vi "Rozbijanie_NMEA_v1.1.vi"() -> ()   [LabVIEW 2014]
uses:
  <vilib>/Instr/_visa.llb/VISA Configure Serial Port (Instr).vi
  <vilib>/robotics/Protocols/NMEA/NMEA API.lvlib
panel:
  out "dane gpsa":T1 {"latitude" format="%#_10g"; "longitiude" format="%#_10g"}
  in  "stop udp":bool
  in  "udp 1":bool
  out "latitude (deg)":dbl format="%#_8g"
  out "longitude (deg)":dbl format="%#_8g"
  out "Cluster":T2 {"Latitude"."DD" format="%#_10g"; "Longitude"."DD" format="%#_10g"}
  out "GPS data":T3 {"oldest read timestamp" format="%^<%.3X\n%x>T"; "latitude (deg)" format="%#_10g"; "longitude (deg)" format="%#_10g"}
  out "f":string
  out "Sekundy 6":dbl
  out "Minuty 6":dbl
  out "Stopnie 6":ext
  out "Sekundy 5":dbl
  out "Minuty 5":dbl
  out "Stopnie 5":ext
  out "Sekundy 4":dbl
  out "Minuty 4":dbl
  out "Stopnie 4":ext
  out "Sekundy 3":dbl
  out "Minuty 3":dbl
  out "Stopnie 3":ext
  in  "stop":bool
  out "return count":u32
  in  "VISA resource name":refnum<visa-resource-name>="COM1"
  out "Sekundy 2":dbl
  out "Minuty 2":dbl
  out "Stopnie 2":ext
  out "Sekundy":dbl
  out "Minuty":dbl
  out "Stopnie":ext
  out "Array":string[](array[string])
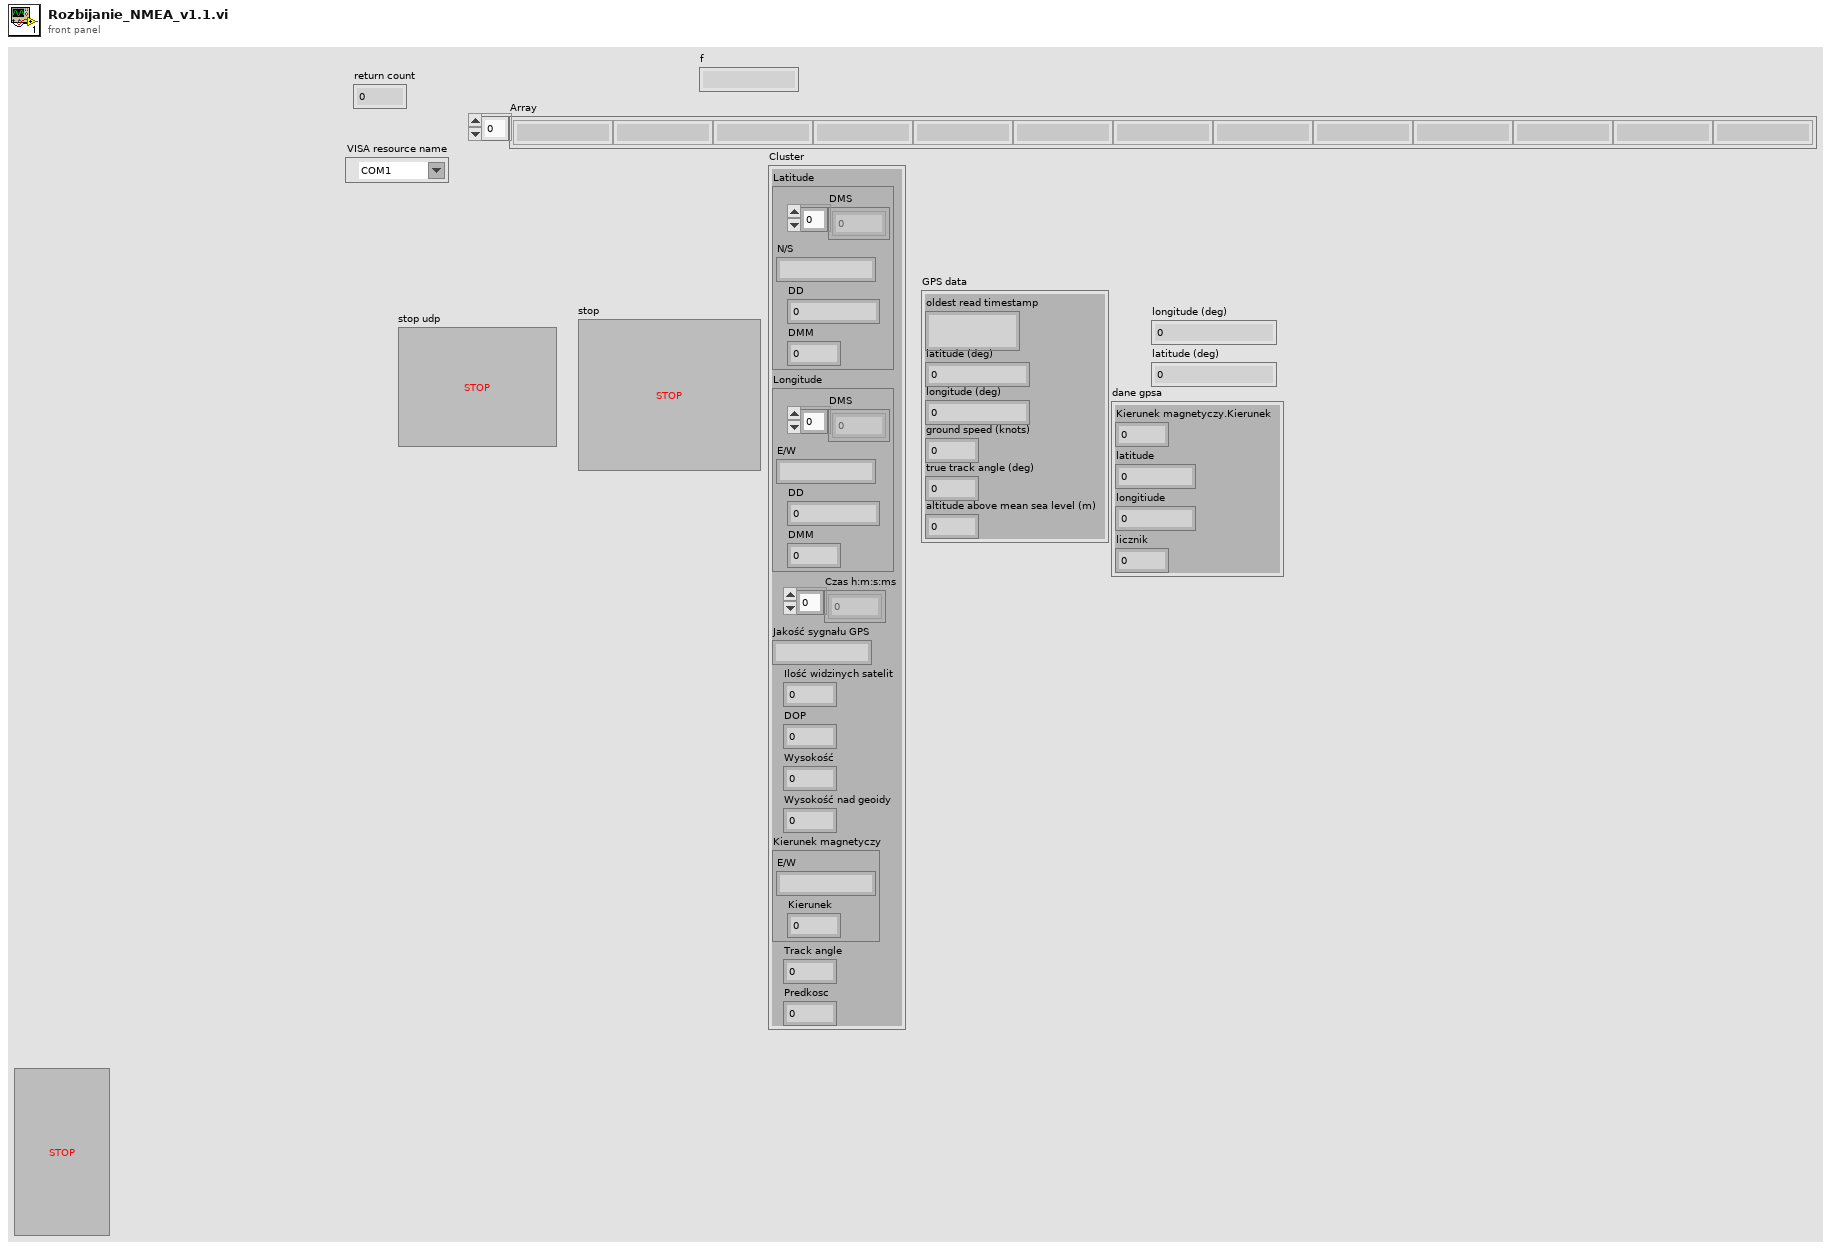
[diagram p1: front panel]
types:
  T1 = cluster{"Kierunek magnetyczy.Kierunek":dbl, "latitude":dbl, "longitiude":dbl, "licznik":dbl}
  T2 = cluster{"Latitude":cluster{"DMS":i32[], "N/S":string, "DD":dbl, "DMM":dbl}, "Longitude":cluster{"DMS":i32[], "E/W":string, "DD":dbl, "DMM":dbl}, "Czas h:m:s:ms":dbl[], "Jakość sygnału GPS":string, "Ilość widzinych satelit":i32, "DOP":dbl, "Wysokość":dbl, "Wysokość nad geoidy":dbl, "Kierunek magnetyczy":cluster{"E/W":string, "Kierunek":dbl}, "Track angle":dbl, "Predkosc":dbl}
  T3 = cluster{"oldest read timestamp":timestamp, "latitude (deg)":dbl, "longitude (deg)":dbl, "ground speed (knots)":dbl, "true track angle (deg)":dbl, "altitude above mean sea level (m)":dbl}
  T4 = cluster{"DMS":i32[], "E/W":string, "DD":dbl, "DMM":dbl}
  T5 = cluster{"DMS":i32[], "N/S":string, "DD":dbl, "DMM":dbl}
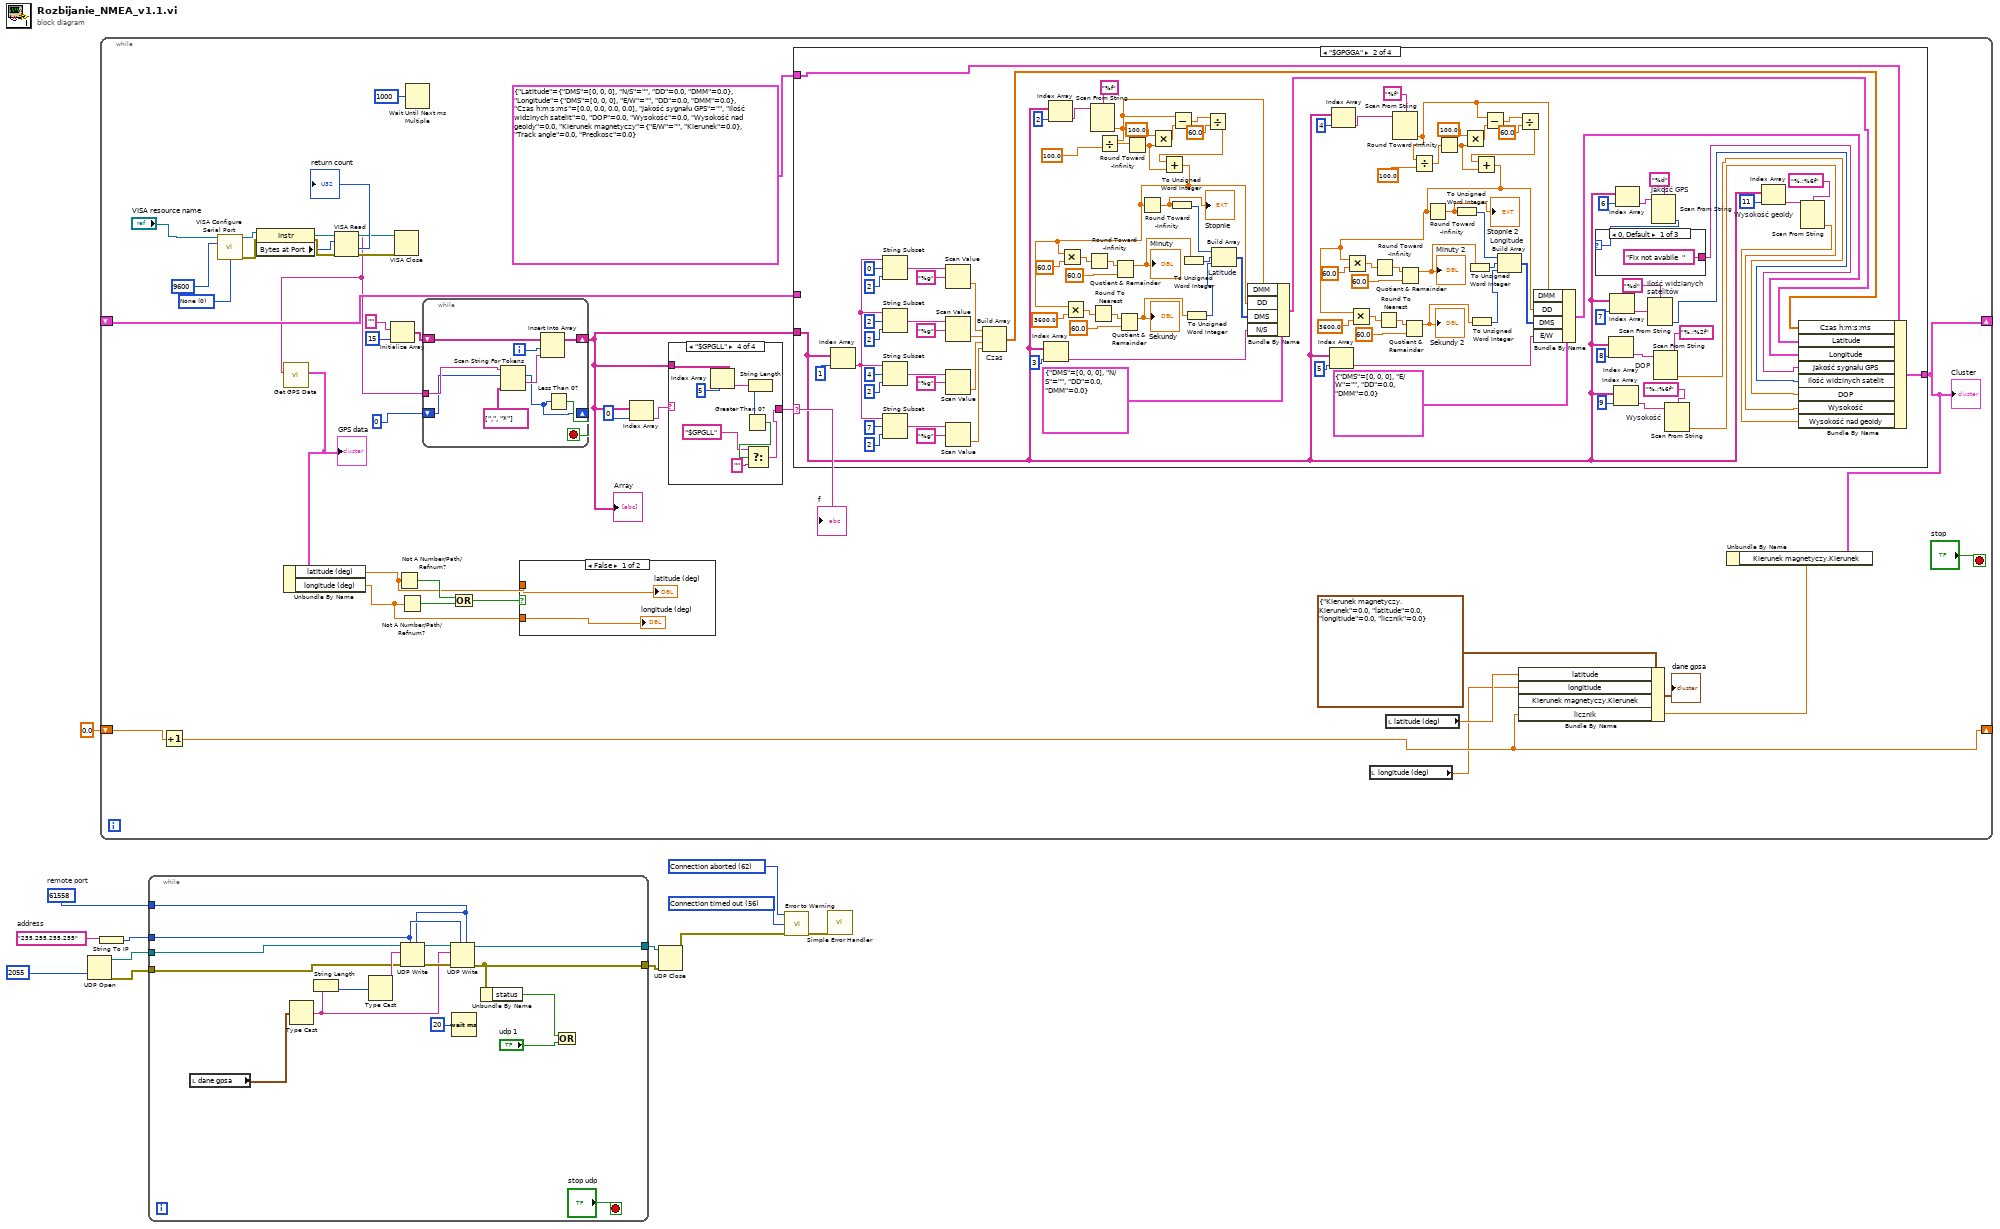
[diagram p0: block diagram]
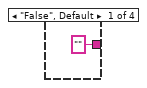
[diagram p3: hidden frame]
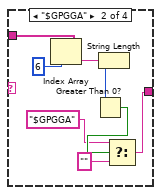
[diagram p4: hidden frame]
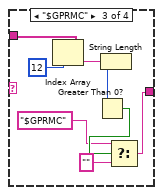
[diagram p5: hidden frame]
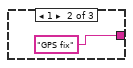
[diagram p7: hidden frame]
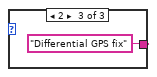
[diagram p8: hidden frame]
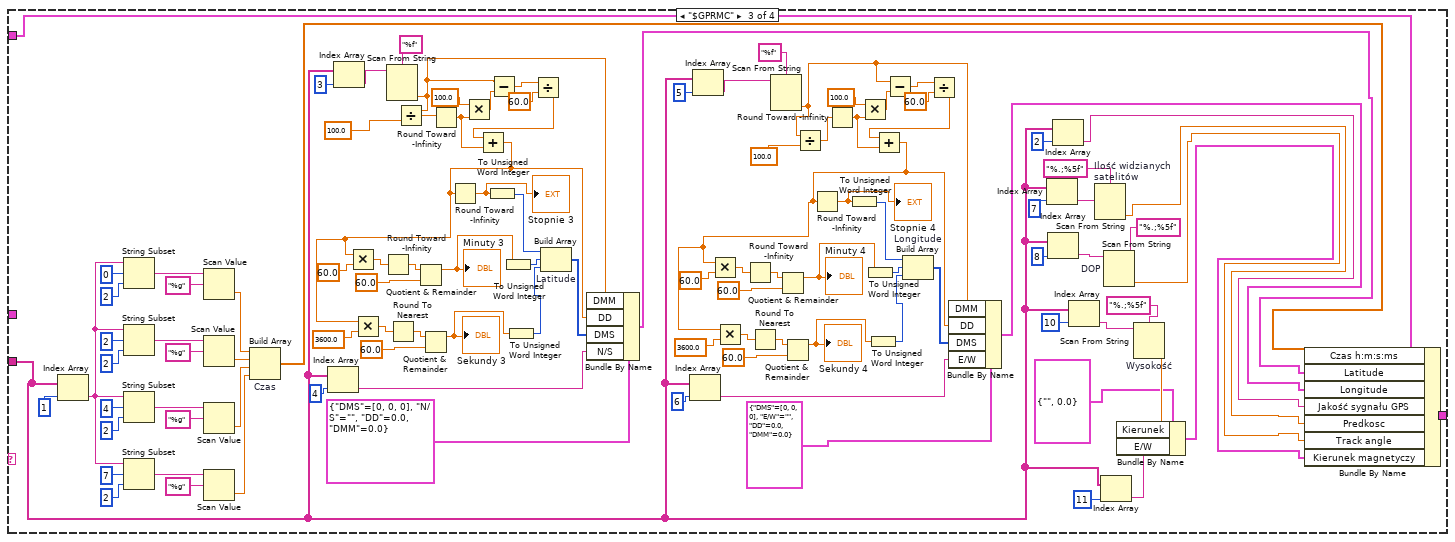
[diagram p9: hidden frame]
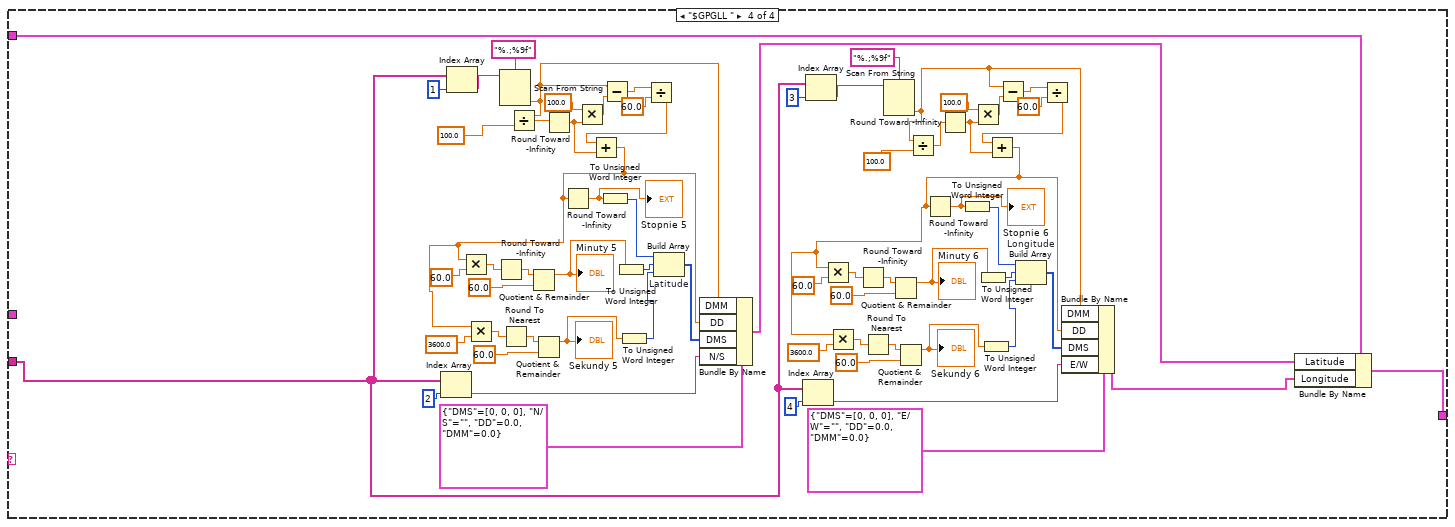
[diagram p10: hidden frame]
diagram:
  w10 = 56 items=["No Error", "Argument Error", "Memory Full", "Out of Zone", "End of File", "File Already Open", "Generic File IO Error", "File Not Found", "File Permission Error", "Disk Full", "Duplicate Path", "Too Many Files Open", "Not Enabled", "Resource File Not Found", "Cannot Add Resource", "Resource Not Found", "Image Not Found", "Image Memory Error", "Pen Does Not Exist", "Config Bad Type", "Config Token Not Found", "Config Parse Error", "Config Memory Error", "Bad External Code Format", "Bad External Code Offset", "External Code Not Present", "Null Window", "Destroy Window Mixup", "Null Menu", "Print Aborted", "Bad Print Record", "Print Driver Error", "Windows Error During Print", "Memory Error During Print", "Print Dialog Error", "Generic Print Error", "Invalid Device Refnum", "Device Not Found", "Device Parameter Error", "Device Unit Error", "Can't Open Device", "Device Call Aborted", "Generic Error", "Cancelled By User", "Object ID Too Low", "Object ID Too High", "Object Not In Heap", "Unknown Heap", "Bad DefProc ID", "DefProc Not In Table", "Message Out Of Range", "Null Method", "Unknown Message", "Manager Call Not Supported", "Bad address", "Connection In progress", "Connection timed out", "Connection is already in progress", "Network attribute not supported", "Network error", "Address in use", "System out of memory", "Connection aborted", "Connection refused", "Connection is not connected", "Connection is already connected", "Connection closed", "Initialize error (interapplication manager)", "Bad occurrence", "Wait on unbound occurrence handler", "Occurrence queue overflow", "Bad path", "Semaphore not signaled", "Unrecognized type (interapplication manager)"] ("3rd Error to Convert")
  w9 = 62 items=["No Error", "Argument Error", "Memory Full", "Out of Zone", "End of File", "File Already Open", "Generic File IO Error", "File Not Found", "File Permission Error", "Disk Full", "Duplicate Path", "Too Many Files Open", "Not Enabled", "Resource File Not Found", "Cannot Add Resource", "Resource Not Found", "Image Not Found", "Image Memory Error", "Pen Does Not Exist", "Config Bad Type", "Config Token Not Found", "Config Parse Error", "Config Memory Error", "Bad External Code Format", "Bad External Code Offset", "External Code Not Present", "Null Window", "Destroy Window Mixup", "Null Menu", "Print Aborted", "Bad Print Record", "Print Driver Error", "Windows Error During Print", "Memory Error During Print", "Print Dialog Error", "Generic Print Error", "Invalid Device Refnum", "Device Not Found", "Device Parameter Error", "Device Unit Error", "Can't Open Device", "Device Call Aborted", "Generic Error", "Cancelled By User", "Object ID Too Low", "Object ID Too High", "Object Not In Heap", "Unknown Heap", "Bad DefProc ID", "DefProc Not In Table", "Message Out Of Range", "Null Method", "Unknown Message", "Manager Call Not Supported", "Bad address", "Connection In progress", "Connection timed out", "Connection is already in progress", "Network attribute not supported", "Network error", "Address in use", "System out of memory", "Connection aborted", "Connection refused", "Connection is not connected", "Connection is already connected", "Connection closed", "Initialize error (interapplication manager)", "Bad occurrence", "Wait on unbound occurrence handler", "Occurrence queue overflow", "Bad path", "Semaphore not signaled", "Unrecognized type (interapplication manager)"] ("1st Error to Convert")
  w4 = u16 61558  # remote port
  w13 = "255.255.255.255"  # address
  n1 = UDP Open(11:u16 2055 ("port")) -> (port=w3:refnum<k16>, 0:w2:errorcluster)  [unwired: 4 in, 1 out]
  n2 = String To IP(1:w13) -> (0:w5:u32)
  n3 = while {
    shift-right: [w23] -> _
    shift-left: _ -> [w29]
    shift-right: [w18] -> _
    shift-left: 0.0 -> [w19]
    stop <- "stop" stop-if-true
    w36 = u16 0 items=["None", "XON/XOFF", "RTS/CTS", "XON/XOFF & RTS/CTS", "DTR/DSR", "XON/XOFF & DTR/DSR"] ("flow control (0:none)")
    n4 = Increment(x=w19) -> (x+1=w18:dbl)
    n5 = call-poly "VISA Configure Serial Port"("VISA resource name"="VISA resource name", "baud rate (9600)"=u32 9600, "flow control (0:none)"=w36) -> ("VISA resource name out"=w40:refnum<visa-resource-name>, "error out"=w39:errorcluster)  [unwired: 11 in]
    n6 = property class="Instr"(reference=w40, error in=w39) -> (reference out=w47:refnum<visa-resource-name>, error out=w46:errorcluster, "Bytes at Port"=w45:u32)
    n7 = VISA Read(VISA resource name=w47, byte count=w45, error in (no error)=w46) -> (VISA resource name out=w43:refnum<visa-resource-name>, read buffer=w28:string, return count=→"return count":u32, error out=w42:errorcluster)
    n8 = call <vilib>:"Get GPS Data.vi"("sensor data"=w28) -> ("GPS data"=w27:T3)  [unwired: 8 in, 2 out]
    "GPS data" <- w27
    n9 = Unbundle By Name(w27) -> ("latitude (deg)"=w17:dbl, "longitude (deg)"=w16:dbl)
    n10 = Initialize Array("", 15 ("dimension size")) -> (w49:string[])
    n11 = VISA Close(VISA resource name=w43, error in (no error)=w42) -> ()  [unwired: 1 out]
    n12 = Not A Number/Path/Refnum?(number/path/refnum=w17) -> (NaN/Path/Refnum?=w26:bool)
    n13 = Not A Number/Path/Refnum?(number/path/refnum=w16) -> (NaN/Path/Refnum?=w25:bool)
    n14 = Wait Until Next ms Multiple(millisecond multiple=u32 1000) -> ()  [unwired: 1 out]
    n15 = while {
      shift-right: [w82] -> w32
      shift-left: w49 -> [w85]
      tunnel: w28 -> [w84]
      shift-right: [w79] -> _
      shift-left: 0 ("token index") -> [w80]
      i -> [w87]
      stop <- w81 stop-if-true
      n16 = Scan String For Tokens(6:string[] [",", "*"] ("delimiters (\\s,\\t,\\r,\\n)"), 8:w80, 9:w84) -> (1:w86:string, 2:w79:i32)  [unwired: 3 in, 2 out]
      n17 = Insert Into Array(array=w85, index=w87, new element=w86) -> (w82:string[])
      n18 = Less Than 0?(x=w79) -> (x < 0?=w81:bool)
    }
    "Array" <- w32
    n19 = Or(x=w26, y=w25) -> (x .or. y?=w24:bool)
    n20 = case shown="False" w24 {
      tunnel: w16 -> [w53 _]
      tunnel: w17 -> [w52 _]
      frame False {
        "longitude (deg)" <- w53
        "latitude (deg)" <- w52
      }
      frame True {
      }
    }
    n21 = Index Array(array=w32, index=0) -> (element=w33:string)
    n22 = case shown="\"$GPGLL\"" w33 {
      tunnel: w32 -> [_ w61 w64 w72]
      tunnel: ["" ("f") w56 w63 w71] -> w31
      frame "False", Default {
      }
      frame "$GPGGA" {
        n23 = Index Array(array=w61, index=6) -> (element=w60:string)
        n24 = String Length(string=w60) -> (length=w59:i32)
        n25 = Greater Than 0?(x=w59) -> (x > 0?=w58:bool)
        n26 = Select(t="$GPGGA", s=w58, f="") -> (s? t:f=w56:string)
      }
      frame "$GPRMC" {
        n27 = Index Array(array=w64, index=12) -> (element=w69:string)
        n28 = String Length(string=w69) -> (length=w68:i32)
        n29 = Greater Than 0?(x=w68) -> (x > 0?=w67:bool)
        n30 = Select(t="$GPRMC", s=w67, f="") -> (s? t:f=w63:string)
      }
      frame "$GPGLL" {
        n31 = Index Array(array=w72, index=5) -> (element=w77:string)
        n32 = String Length(string=w77) -> (length=w76:i32)
        n33 = Greater Than 0?(x=w76) -> (x > 0?=w75:bool)
        n34 = Select(t="$GPGLL", s=w75, f="") -> (s? t:f=w71:string)
      }
    }
    "f" <- w31
    n35 = case shown="\"$GPGGA\"" w31 {
      tunnel: w32 -> [_ w122 w215 w313]
      tunnel: [w88 w90 w210 w315] -> w23
      tunnel: T2 {"Latitude"={"DMS"=[0, 0, 0], "N/S"="", "DD"=0.0, "DMM"=0.0}, "Longitude"={"DMS"=[0, 0, 0], "E/W"="", "DD"=0.0, "DMM"=0.0}, "Czas h:m:s:ms"=[0.0, 0.0, 0.0, 0.0], "Jakość sygnału GPS"="", "Ilość widzinych satelit"=0, "DOP"=0.0, "Wysokość"=0.0, "Wysokość nad geoidy"=0.0, "Kierunek magnetyczy"={"E/W"="", "Kierunek"=0.0}, "Track angle"=0.0, "Predkosc"=0.0} -> [_ w89 w211 w316]
      tunnel: w29 -> [w88 _ _ _]
      frame "False", Default {
      }
      frame "$GPGGA" {
        n36 = Index Array(array=w122, index=1) -> (element=w182:string)
        n37 = String Subset(string=w182, offset (0)=0, length (rest)=2 ("length (rest)")) -> (substring=w196:string)
        n38 = String Subset(string=w182, offset (0)=2, length (rest)=2 ("length (rest)")) -> (substring=w192:string)
        n39 = String Subset(string=w182, offset (0)=4, length (rest)=2 ("length (rest)")) -> (substring=w188:string)
        n40 = String Subset(string=w182, offset (0)=7, length (rest)=2 ("length (rest)")) -> (substring=w184:string)
        n41 = Scan Value(string=w196, format string="%g") -> (value=w181:dbl)  [unwired: 1 in, 1 out]
        n42 = Scan Value(string=w192, format string="%g") -> (value=w180:dbl)  [unwired: 1 in, 1 out]
        n43 = Scan Value(string=w188, format string="%g") -> (value=w179:dbl)  [unwired: 1 in, 1 out]
        n44 = Scan Value(string=w184, format string="%g") -> (value=w178:dbl)  [unwired: 1 in, 1 out]
        n45 = Build Array "Czas"(w181, w180, w179, w178) -> (w111:dbl[])
        n46 = Index Array(array=w122, index=3) -> (element=w159:string)
        n47 = Index Array(array=w122, index=2) -> (element=w175:string)
        n48 = Scan From String(format string="%f", input string=w175) -> (output 1=w106:dbl)  [unwired: 3 in, 3 out]
        n49 = Divide(x=w106, y=100.0) -> (x/y=w109:dbl)
        n50 = Round Toward -Infinity(1:w109) -> (0:w103:dbl)
        n51 = Multiply(x=100.0, y=w103) -> (x*y=w107:dbl)
        n52 = Subtract(x=w106, y=w107) -> (x-y=w105:dbl)
        n53 = Divide(x=w105, y=60.0) -> (x/y=w102:dbl)
        n54 = Add(x=w102, y=w103) -> (x+y=w101:dbl)
        n55 = Multiply(x=w101, y=60.0) -> (x*y=w172:dbl)
        n56 = Multiply(x=w101, y=3600.0) -> (x*y=w168:dbl)
        n57 = Round Toward -Infinity(1:w172) -> (0:w171:dbl)
        n58 = Round To Nearest(number=w168) -> (nearest integer value=w167:dbl)
        n59 = Quotient & Remainder(x=w171, y=60.0) -> (x-y*floor(x/y)=w163:dbl)  [unwired: 1 out]
        "Minuty" <- w163
        n60 = Quotient & Remainder(x=w167, y=60.0) -> (x-y*floor(x/y)=w161:dbl)  [unwired: 1 out]
        "Sekundy" <- w161
        n61 = Round Toward -Infinity(1:w101) -> (0:w137:dbl)
        "Stopnie" <- w137
        n62 = To Unsigned Word Integer(number=w137) -> (unsigned 16bit integer=w165:u16)
        n63 = To Unsigned Word Integer(number=w163) -> (unsigned 16bit integer=w164:u16)
        n64 = To Unsigned Word Integer(number=w161) -> (unsigned 16bit integer=w162:u16)
        n65 = Build Array "Latitude"(w165, w164, w162) -> (w160:u16[])
        n66 = Bundle By Name(cluster=T5 {"DMS"=[0, 0, 0], "N/S"="", "DD"=0.0, "DMM"=0.0}, "DMM"=w106, "DD"=w101, "DMS"=w160, "N/S"=w159) -> (w112:T5)
        n67 = Index Array(array=w122, index=5) -> (element=w140:string)
        n68 = Index Array(array=w122, index=4) -> (element=w156:string)
        n69 = Scan From String(format string="%f", input string=w156) -> (output 1=w91:dbl)  [unwired: 3 in, 3 out]
        n70 = Divide(x=w91, y=100.0) -> (x/y=w93:dbl)
        n71 = Round Toward -Infinity(1:w93) -> (0:w99:dbl)
        n72 = Multiply(x=100.0, y=w99) -> (x*y=w96:dbl)
        n73 = Subtract(x=w91, y=w96) -> (x-y=w97:dbl)
        n74 = Divide(x=w97, y=60.0) -> (x/y=w100:dbl)
        n75 = Add(x=w100, y=w99) -> (x+y=w92:dbl)
        n76 = Multiply(x=w92, y=60.0) -> (x*y=w153:dbl)
        n77 = Multiply(x=w92, y=3600.0) -> (x*y=w149:dbl)
        n78 = Round Toward -Infinity(1:w153) -> (0:w152:dbl)
        n79 = Round To Nearest(number=w149) -> (nearest integer value=w148:dbl)
        n80 = Quotient & Remainder(x=w152, y=60.0) -> (x-y*floor(x/y)=w144:dbl)  [unwired: 1 out]
        "Minuty 2" <- w144
        n81 = Quotient & Remainder(x=w148, y=60.0) -> (x-y*floor(x/y)=w142:dbl)  [unwired: 1 out]
        "Sekundy 2" <- w142
        n82 = Round Toward -Infinity(1:w92) -> (0:w136:dbl)
        "Stopnie 2" <- w136
        n83 = To Unsigned Word Integer(number=w136) -> (unsigned 16bit integer=w146:u16)
        n84 = To Unsigned Word Integer(number=w144) -> (unsigned 16bit integer=w145:u16)
        n85 = To Unsigned Word Integer(number=w142) -> (unsigned 16bit integer=w143:u16)
        n86 = Build Array "Longitude"(w146, w145, w143) -> (w141:u16[])
        n87 = Bundle By Name(cluster=T4 {"DMS"=[0, 0, 0], "E/W"="", "DD"=0.0, "DMM"=0.0}, "DMM"=w91, "DD"=w92, "DMS"=w141, "E/W"=w140) -> (w113:T4)
        n88 = Index Array(array=w122, index=8) -> (element=w126:string)
        n89 = Index Array(array=w122, index=7) -> (element=w130:string)
        n90 = Index Array(array=w122, index=9) -> (element=w124:string)
        n91 = Index Array(array=w122, index=6) -> (element=w134:string)
        n92 = Scan From String "Ilość widzianych satelitów"(format string="%d", input string=w130) -> (output 1=w115:i32)  [unwired: 3 in, 3 out]
        n93 = Scan From String "Jakość GPS"(format string="%d", input string=w134) -> (output 1=w132:i32)  [unwired: 3 in, 3 out]
        n94 = case shown="0, Default" w132 {
          tunnel: ["Fix not avabile  " "GPS fix" "Differential GPS fix"] -> w114
          frame 0, Default {
          }
          frame 1 {
          }
          frame 2 {
          }
        }
        n95 = Scan From String "DOP"(format string="%.;%2f", input string=w126) -> (output 1=w116:dbl)  [unwired: 3 in, 3 out]
        n96 = Scan From String "Wysokość"(format string="%.;%6f", input string=w124) -> (output 1=w117:dbl)  [unwired: 3 in, 3 out]
        n97 = Index Array(array=w122, index=11) -> (element=w120:string)
        n98 = Scan From String "Wysokość geoidy"(format string="%,;%6f", input string=w120) -> (output 1=w118:dbl)  [unwired: 3 in, 3 out]
        n99 = Bundle By Name(cluster=w89, "Czas h:m:s:ms"=w111, "Latitude"=w112, "Longitude"=w113, "Jakość sygnału GPS"=w114, "Ilość widzinych satelit"=w115, "DOP"=w116, "Wysokość"=w117, "Wysokość nad geoidy"=w118) -> (w90:T2)
      }
      frame "$GPRMC" {
        n100 = Index Array(array=w215, index=1) -> (element=w237:string)
        n101 = String Subset(string=w237, offset (0)=0, length (rest)=2 ("length (rest)")) -> (substring=w223:string)
        n102 = String Subset(string=w237, offset (0)=2, length (rest)=2 ("length (rest)")) -> (substring=w227:string)
        n103 = String Subset(string=w237, offset (0)=4, length (rest)=2 ("length (rest)")) -> (substring=w231:string)
        n104 = String Subset(string=w237, offset (0)=7, length (rest)=2 ("length (rest)")) -> (substring=w235:string)
        n105 = Scan Value(string=w223, format string="%g") -> (value=w238:dbl)  [unwired: 1 in, 1 out]
        n106 = Scan Value(string=w227, format string="%g") -> (value=w239:dbl)  [unwired: 1 in, 1 out]
        n107 = Scan Value(string=w231, format string="%g") -> (value=w240:dbl)  [unwired: 1 in, 1 out]
        n108 = Scan Value(string=w235, format string="%g") -> (value=w241:dbl)  [unwired: 1 in, 1 out]
        n109 = Build Array "Czas"(w238, w239, w240, w241) -> (w209:dbl[])
        n110 = Index Array(array=w215, index=4) -> (element=w259:string)
        n111 = Index Array(array=w215, index=3) -> (element=w244:string)
        n112 = Scan From String(format string="%f", input string=w244) -> (output 1=w296:dbl)  [unwired: 3 in, 3 out]
        n113 = Divide(x=w296, y=100.0) -> (x/y=w293:dbl)
        n114 = Round Toward -Infinity(1:w293) -> (0:w299:dbl)
        n115 = Multiply(x=100.0, y=w299) -> (x*y=w295:dbl)
        n116 = Subtract(x=w296, y=w295) -> (x-y=w297:dbl)
        n117 = Divide(x=w297, y=60.0) -> (x/y=w300:dbl)
        n118 = Add(x=w300, y=w299) -> (x+y=w301:dbl)
        n119 = Multiply(x=w301, y=60.0) -> (x*y=w247:dbl)
        n120 = Multiply(x=w301, y=3600.0) -> (x*y=w251:dbl)
        n121 = Round Toward -Infinity(1:w247) -> (0:w248:dbl)
        n122 = Round To Nearest(number=w251) -> (nearest integer value=w252:dbl)
        n123 = Quotient & Remainder(x=w248, y=60.0) -> (x-y*floor(x/y)=w255:dbl)  [unwired: 1 out]
        "Minuty 3" <- w255
        n124 = Quotient & Remainder(x=w252, y=60.0) -> (x-y*floor(x/y)=w257:dbl)  [unwired: 1 out]
        "Sekundy 3" <- w257
        n125 = Round Toward -Infinity(1:w301) -> (0:w280:dbl)
        "Stopnie 3" <- w280
        n126 = To Unsigned Word Integer(number=w280) -> (unsigned 16bit integer=w253:u16)
        n127 = To Unsigned Word Integer(number=w255) -> (unsigned 16bit integer=w254:u16)
        n128 = To Unsigned Word Integer(number=w257) -> (unsigned 16bit integer=w256:u16)
        n129 = Build Array "Latitude"(w253, w254, w256) -> (w258:u16[])
        n130 = Bundle By Name(cluster=T5 {"DMS"=[0, 0, 0], "N/S"="", "DD"=0.0, "DMM"=0.0}, "DMM"=w296, "DD"=w301, "DMS"=w258, "N/S"=w259) -> (w208:T5)
        n131 = Index Array(array=w215, index=6) -> (element=w277:string)
        n132 = Index Array(array=w215, index=5) -> (element=w213:string)
        n133 = Scan From String(format string="%f", input string=w213) -> (output 1=w212:dbl)  [unwired: 3 in, 3 out]
        n134 = Divide(x=w212, y=100.0) -> (x/y=w309:dbl)
        n135 = Round Toward -Infinity(1:w309) -> (0:w303:dbl)
        n136 = Multiply(x=100.0, y=w303) -> (x*y=w306:dbl)
        n137 = Subtract(x=w212, y=w306) -> (x-y=w305:dbl)
        n138 = Divide(x=w305, y=60.0) -> (x/y=w302:dbl)
        n139 = Add(x=w302, y=w303) -> (x+y=w310:dbl)
        n140 = Multiply(x=w310, y=60.0) -> (x*y=w264:dbl)
        n141 = Multiply(x=w310, y=3600.0) -> (x*y=w268:dbl)
        n142 = Round Toward -Infinity(1:w264) -> (0:w265:dbl)
        n143 = Round To Nearest(number=w268) -> (nearest integer value=w269:dbl)
        n144 = Quotient & Remainder(x=w265, y=60.0) -> (x-y*floor(x/y)=w273:dbl)  [unwired: 1 out]
        "Minuty 4" <- w273
        n145 = Quotient & Remainder(x=w269, y=60.0) -> (x-y*floor(x/y)=w275:dbl)  [unwired: 1 out]
        "Sekundy 4" <- w275
        n146 = Round Toward -Infinity(1:w310) -> (0:w281:dbl)
        "Stopnie 4" <- w281
        n147 = To Unsigned Word Integer(number=w281) -> (unsigned 16bit integer=w271:u16)
        n148 = To Unsigned Word Integer(number=w273) -> (unsigned 16bit integer=w272:u16)
        n149 = To Unsigned Word Integer(number=w275) -> (unsigned 16bit integer=w274:u16)
        n150 = Build Array "Longitude"(w271, w272, w274) -> (w276:u16[])
        n151 = Bundle By Name(cluster=T4 {"DMS"=[0, 0, 0], "E/W"="", "DD"=0.0, "DMM"=0.0} ("Cluster 2"), "DMM"=w212, "DD"=w310, "DMS"=w276, "E/W"=w277) -> (w207:T4)
        n152 = Index Array(array=w215, index=7) -> (element=w284:string)
        n153 = Index Array(array=w215, index=8) -> (element=w288:string)
        n154 = Index Array(array=w215, index=2) -> (element=w206:string)
        n155 = Index Array(array=w215, index=10) -> (element=w290:string)
        n156 = Scan From String "Ilość widzianych satelitów"(format string="%.;%5f", input string=w284) -> (output 1=w205:dbl)  [unwired: 3 in, 3 out]
        n157 = Index Array(array=w215, index=11) -> (element=w216:string)
        n158 = Scan From String "DOP"(format string="%.;%5f", input string=w288) -> (output 1=w204:dbl)  [unwired: 3 in, 3 out]
        n159 = Scan From String "Wysokość"(format string="%.;%5f", input string=w290) -> (output 1=w218:dbl)  [unwired: 3 in, 3 out]
        n160 = Bundle By Name(cluster=cluster{"E/W":string, "Kierunek":dbl} {"E/W"="", "Kierunek"=0.0}, "Kierunek"=w218, "E/W"=w216) -> (w203:cluster{"E/W":string, "Kierunek":dbl})
        n161 = Bundle By Name(cluster=w211, "Czas h:m:s:ms"=w209, "Latitude"=w208, "Longitude"=w207, "Jakość sygnału GPS"=w206, "Predkosc"=w205, "Track angle"=w204, "Kierunek magnetyczy"=w203) -> (w210:T2)
      }
      frame "$GPGLL " {
        n162 = Index Array(array=w313, index=2) -> (element=w335:string)
        n163 = Index Array(array=w313, index=1) -> (element=w320:string)
        n164 = Scan From String(format string="%.;%9f", input string=w320) -> (output 1=w363:dbl)  [unwired: 3 in, 3 out]
        n165 = Divide(x=w363, y=100.0) -> (x/y=w360:dbl)
        n166 = Round Toward -Infinity(1:w360) -> (0:w366:dbl)
        n167 = Multiply(x=100.0, y=w366) -> (x*y=w362:dbl)
        n168 = Subtract(x=w363, y=w362) -> (x-y=w364:dbl)
        n169 = Divide(x=w364, y=60.0) -> (x/y=w367:dbl)
        n170 = Add(x=w367, y=w366) -> (x+y=w314:dbl)
        n171 = Multiply(x=w314, y=60.0) -> (x*y=w323:dbl)
        n172 = Multiply(x=w314, y=3600.0) -> (x*y=w327:dbl)
        n173 = Round Toward -Infinity(1:w323) -> (0:w324:dbl)
        n174 = Round To Nearest(number=w327) -> (nearest integer value=w328:dbl)
        n175 = Quotient & Remainder(x=w324, y=60.0) -> (x-y*floor(x/y)=w331:dbl)  [unwired: 1 out]
        "Minuty 5" <- w331
        n176 = Quotient & Remainder(x=w328, y=60.0) -> (x-y*floor(x/y)=w333:dbl)  [unwired: 1 out]
        "Sekundy 5" <- w333
        n177 = Round Toward -Infinity(1:w314) -> (0:w357:dbl)
        "Stopnie 5" <- w357
        n178 = To Unsigned Word Integer(number=w357) -> (unsigned 16bit integer=w329:u16)
        n179 = To Unsigned Word Integer(number=w331) -> (unsigned 16bit integer=w330:u16)
        n180 = To Unsigned Word Integer(number=w333) -> (unsigned 16bit integer=w332:u16)
        n181 = Build Array "Latitude"(w329, w330, w332) -> (w334:u16[])
        n182 = Bundle By Name(cluster=T5 {"DMS"=[0, 0, 0], "N/S"="", "DD"=0.0, "DMM"=0.0}, "DMM"=w363, "DD"=w314, "DMS"=w334, "N/S"=w335) -> (w311:T5)
        n183 = Index Array(array=w313, index=4) -> (element=w354:string)
        n184 = Index Array(array=w313, index=3) -> (element=w338:string)
        n185 = Scan From String(format string="%.;%9f", input string=w338) -> (output 1=w377:dbl)  [unwired: 3 in, 3 out]
        n186 = Divide(x=w377, y=100.0) -> (x/y=w375:dbl)
        n187 = Round Toward -Infinity(1:w375) -> (0:w369:dbl)
        n188 = Multiply(x=100.0, y=w369) -> (x*y=w372:dbl)
        n189 = Subtract(x=w377, y=w372) -> (x-y=w371:dbl)
        n190 = Divide(x=w371, y=60.0) -> (x/y=w368:dbl)
        n191 = Add(x=w368, y=w369) -> (x+y=w376:dbl)
        n192 = Multiply(x=w376, y=60.0) -> (x*y=w341:dbl)
        n193 = Multiply(x=w376, y=3600.0) -> (x*y=w345:dbl)
        n194 = Round Toward -Infinity(1:w341) -> (0:w342:dbl)
        n195 = Round To Nearest(number=w345) -> (nearest integer value=w346:dbl)
        n196 = Quotient & Remainder(x=w342, y=60.0) -> (x-y*floor(x/y)=w350:dbl)  [unwired: 1 out]
        "Minuty 6" <- w350
        n197 = Quotient & Remainder(x=w346, y=60.0) -> (x-y*floor(x/y)=w352:dbl)  [unwired: 1 out]
        "Sekundy 6" <- w352
        n198 = Round Toward -Infinity(1:w376) -> (0:w358:dbl)
        "Stopnie 6" <- w358
        n199 = To Unsigned Word Integer(number=w358) -> (unsigned 16bit integer=w348:u16)
        n200 = To Unsigned Word Integer(number=w350) -> (unsigned 16bit integer=w349:u16)
        n201 = To Unsigned Word Integer(number=w352) -> (unsigned 16bit integer=w351:u16)
        n202 = Build Array "Longitude"(w348, w349, w351) -> (w353:u16[])
        n203 = Bundle By Name(cluster=T4 {"DMS"=[0, 0, 0], "E/W"="", "DD"=0.0, "DMM"=0.0}, "DMM"=w377, "DD"=w376, "DMS"=w353, "E/W"=w354) -> (w312:T4)
        n204 = Bundle By Name(cluster=w316, "Latitude"=w311, "Longitude"=w312) -> (w315:T2)
      }
    }
    "Cluster" <- w23
    n205 = local read "longitude (deg)"() -> (w14:dbl)
    n206 = local read "latitude (deg)"() -> (w15:dbl)
    n207 = Unbundle By Name(w23) -> ("Kierunek magnetyczy.Kierunek"=w21:dbl)
    n208 = Bundle By Name(cluster=T1 {"Kierunek magnetyczy.Kierunek"=0.0, "latitude"=0.0, "longitiude"=0.0, "licznik"=0.0} ("input cluster"), "latitude"=w15, "longitiude"=w14, "Kierunek magnetyczy.Kierunek"=w21, "licznik"=w18) -> (→"dane gpsa":T1)
  }
  n209 = while {
    tunnel: [w385] -> w7
    tunnel: [w384] -> w6
    tunnel: w5 -> [w383]
    tunnel: w4 -> [w382]
    tunnel: w3 -> [w381]
    tunnel: w2 -> [w380]
    stop <- "stop udp" stop-if-true
    n210 = local read "dane gpsa"() -> (w379:T1)
    n211 = Type Cast(x=w379) -> (*(type *) &x=w390:string)  [unwired: 1 out]
    n212 = String Length(string=w390) -> (length=w389:i32)
    n213 = Type Cast(x=w389) -> (*(type *) &x=w388:string)  [unwired: 1 out]
    n214 = UDP Write(address=w383, port or service name=w382, connection ID=w381, data in=w388, 8:w380) -> (error out=w391:errorcluster, 3:w386:refnum<k16>)  [unwired: 1 in]
    n215 = UDP Write(address=w383, port or service name=w382, connection ID=w386, data in=w390, 8:w391) -> (error out=w384:errorcluster, 3:w385:refnum<k16>)  [unwired: 1 in]
    n216 = Wait (ms)(milliseconds to wait=u32 20) -> ()  [unwired: 1 out]
    n217 = Unbundle By Name(w384) -> ("status"=w393:bool)
    n218 = Or(x=w393, y="udp 1") -> ()  [unwired: 1 out]
  }
  n219 = UDP Close(connection ID=w7, 8:w6) -> (error out=w8:errorcluster)  [unwired: 1 out]
  n220 = call <vilib>:"Error to Warning.vi"("1st Error to Convert"=w9, "3rd Error to Convert"=w10, "error in"=w8) -> ("warning out"=w11:errorcluster)  [unwired: 3 in, 9 out]
  n221 = call <vilib>:"Simple Error Handler.vi"("error in (no error)"=w11) -> ()  [unwired: 1 in, 8 out]
